vi "Calculate Desired States.vi"(8 "error in (no error)":errorcluster, 10 "Vessel In":refnum<class "Vessel.lvclass">, 11 "CJ Oculus Rift Guidance in":refnum<class "Oculus Rift Guidance.lvclass">) -> (0 "error out":errorcluster, 2 "Vessel Out":refnum<class "Vessel.lvclass">, 3 "CJ Oculus Rift Guidance out":refnum<class "Oculus Rift Guidance.lvclass">)   [LabVIEW 2014, in "Guidance Library.lvlib" / "Oculus Rift Guidance.lvclass"]
uses:
  Oculus Rift Guidance.lvclass
  ROV/Vessel.lvclass
  <vilib>/Analysis/Matrix/Datatypes/RealMatrix.ctl
  <vilib>/Analysis/baseanly.llb/A x Vector.vi
  Library/Kinematics/J_euler.vi
  Reference Models/Reference Model Joystick.vi
  Library/Integrator/Integrator trapez vector.vi
  Supervisor/Supervisor.lvclass
  <vilib>/Analysis/NI_AALBase.lvlib
  <vilib>/Analysis/Matrix/NI_Matrix.lvlib
panel:
  in  "Reset 0 Pos":bool
  in  "reset":bool
  in  "reset init pos":bool
  out "a 3":dbl(graph)
  out "a 2":dbl(graph)
  out "a":dbl(graph)
  in  "T 3":T1=[[0.0, -1.0, 0.0, 0.0, 0.0, 0.0], [-1.0, 0.0, 0.0, 0.0, 0.0, 0.0], [0.0, 0.0, 0.0, 0.0, 0.0, 0.0], [0.0, 0.0, 0.0, 0.0, 0.0, 0.0], [0.0, 0.0, 0.0, 0.0, 0.0, 0.0], [0.0, 0.0, 0.0, 0.0, 0.0, -1.0]]
  out "Nu_max":dbl[](array[numeric])
  out "yaw":cluster{"Numeric":dbl, dbl}(graph)
  out "sway":cluster{"Numeric":dbl, dbl}(graph)
  out "Surge":cluster{"Numeric":dbl, dbl}(graph)
  in  "Delta":T1=[[1.0, 0.0, 0.0, 0.0, 0.0, 0.0], [1.0, 0.0, 0.0, 0.0, 0.0, 0.0], [1.0, 0.0, 0.0, 0.0, 0.0, 0.0], [1.0, 0.0, 0.0, 0.0, 0.0, 0.0], [1.0, 0.0, 0.0, 0.0, 0.0, 0.0], [1.0, 0.0, 0.0, 0.0, 0.0, 0.0]]
  in  "Omega":T1=[[0.8, 0.0, 0.0, 0.0, 0.0, 0.0], [0.8, 0.0, 0.0, 0.0, 0.0, 0.0], [0.8, 0.0, 0.0, 0.0, 0.0, 0.0], [0.8, 0.0, 0.0, 0.0, 0.0, 0.0], [0.8, 0.0, 0.0, 0.0, 0.0, 0.0], [0.8, 0.0, 0.0, 0.0, 0.0, 0.0]]
  in  "OR Response":u16=1
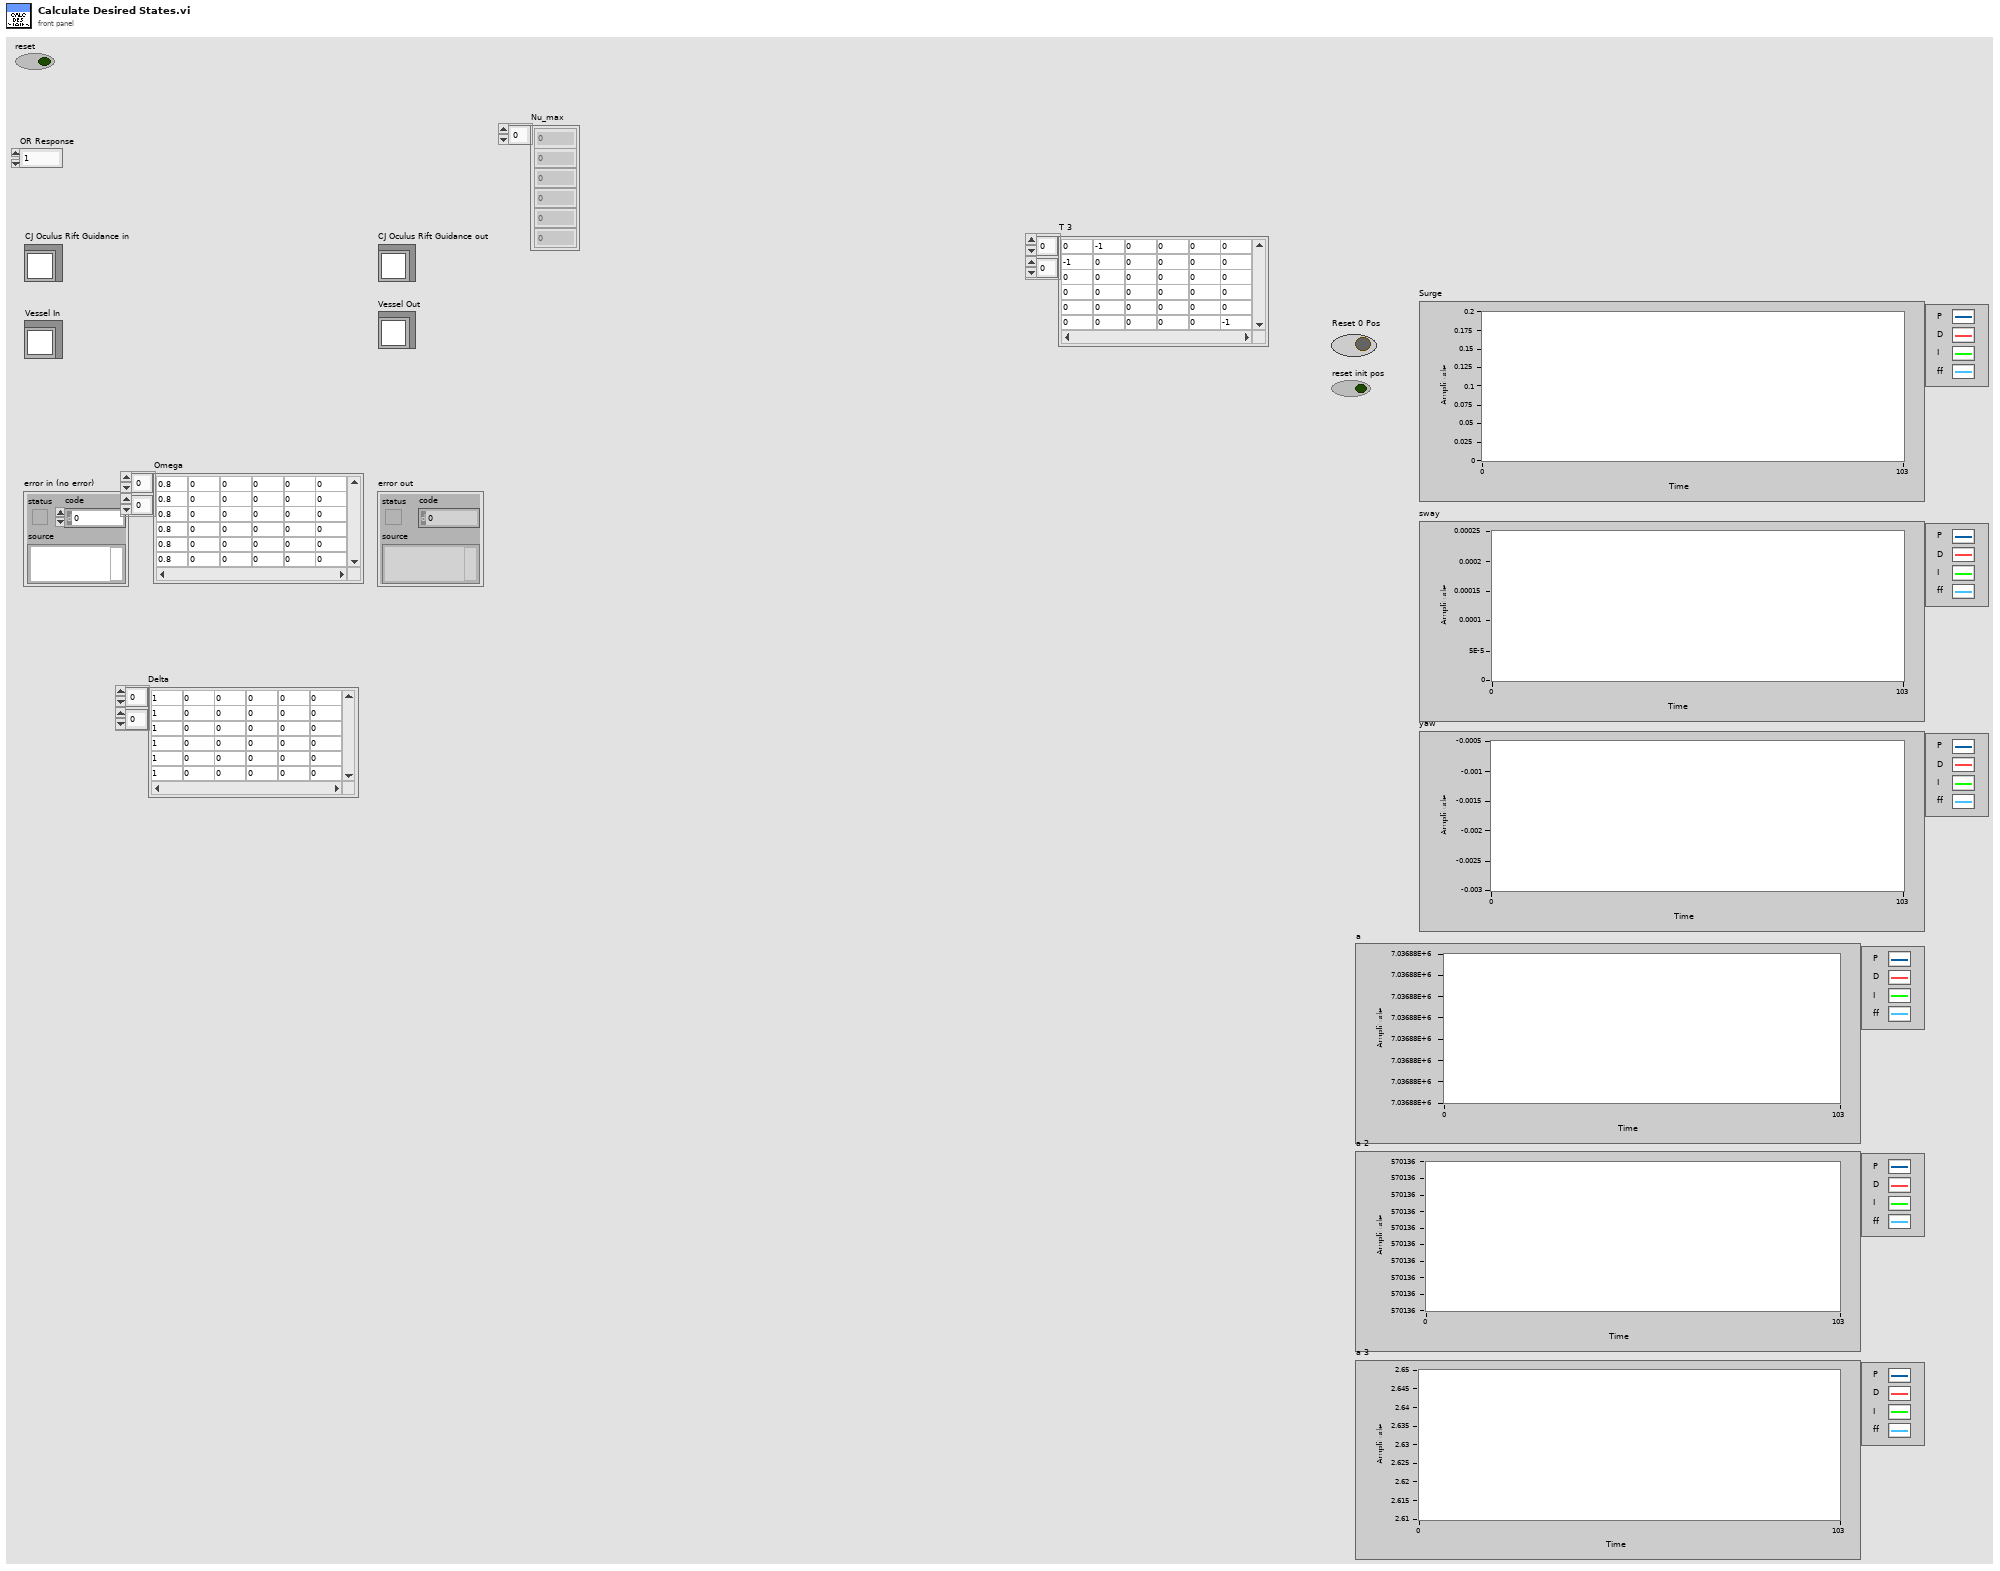
[diagram p1: front panel]
types:
  T1 = typedef "NI_Matrix.lvlib/RealMatrix.ctl" = dbl[][]
  T2 = cluster{"Measured":cluster{"Eta":dbl[], "Nu":dbl[], "Eta Dot":dbl[], "Nu Dot":dbl[]}, "Estimated":cluster{"Eta":dbl[], "Nu":dbl[], "Eta Dot":dbl[], "Nu Dot":dbl[]}, "Desired":cluster{"Eta":dbl[], "Nu":dbl[], "Eta Dot":dbl[], "Nu Dot":dbl[]}, "Previous Desired":cluster{"Eta":dbl[], "Nu":dbl[], "Eta Dot":dbl[], "Nu Dot":dbl[]}, "tau":dbl[], "Altitude":cluster{"Measured":dbl, "Estimated":dbl, "Desired":dbl, "Previous Desired":dbl, "Approximated":dbl, "grad F":dbl[]}, "rpm":dbl[], "Attitude":cluster{"Theta Measured":dbl[], "Theta Estimated":dbl[], "Omega Measured":dbl[], "Omega Estimated":dbl[], "Gyro Bias":dbl[]}}
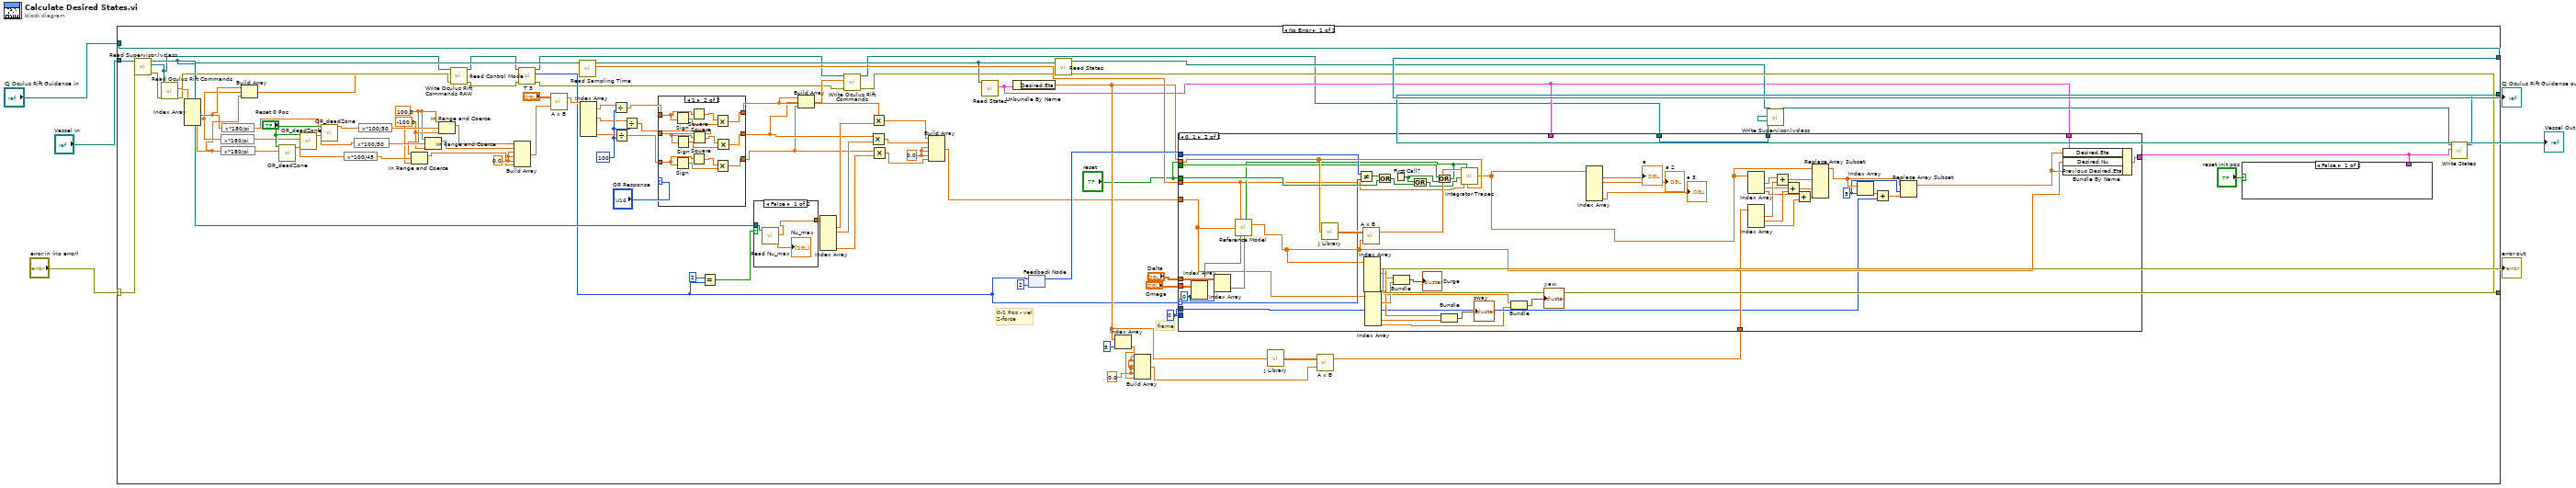
[diagram p0: block diagram]
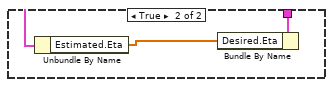
[diagram p2: hidden frame]
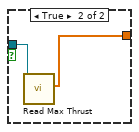
[diagram p3: hidden frame]
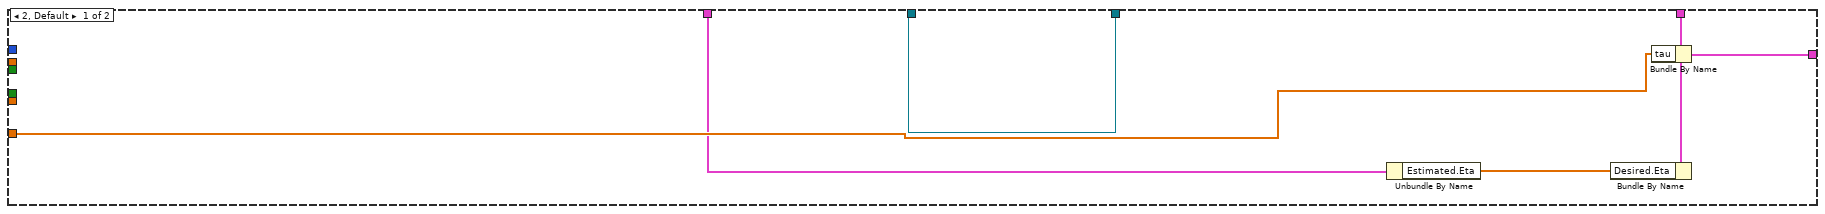
[diagram p4: hidden frame]
diagram:
  n1 = case shown="No Error" "error in (no error)" {
    selector: "error in (no error)" -> [w89 w172]
    tunnel: [w58 w172] -> w2
    tunnel: [w74 w171] -> w4
    tunnel: "CJ Oculus Rift Guidance in" -> [w74 w171]
    tunnel: "Vessel In" -> [w75 w170]
    tunnel: [w67 w170] -> w3
    frame No Error {
      w23 = 100.0 ("upper limit")
      w22 = -100.0 ("lower limit")
      w50 = 0.0
      w65 = 0.0 ("element")
      w66 = u16 0 ("Frame Mode")
      w82 = 0.0
      w88 = 100
      # "frame"
      # "0-1 Pos - vel\n2-force"
      n2 = call "Read Supervisor.lvclass.vi"("error in (no error)"=w89, "Vessel in"=w75) -> ("error out"=w90:errorcluster, "Supervisor.lvclass"=w16:refnum<class "Supervisor.lvclass">, "Vessel out"=w52:refnum<class "Vessel.lvclass">)  [unwired: 7 in]
      n3 = call-dynamic "Read Oculus Rift Commands.vi"("error in (no error)"=w90, "Supervisor in"=w16) -> ("error out"=w17:errorcluster, "Oculus Rift Commands"=w21:dbl[])  [unwired: 7 in, 1 out]
      n4 = Index Array(array=w21) -> (element #2=w9:dbl, element #3=w8:dbl, element #4=w7:dbl)  [unwired: 4 in, 1 out]
      n5 = expression code="x*180/pi"(w8) -> (w31:dbl)
      n6 = expression code="x*180/pi"(w7) -> (w30:dbl)
      n7 = expression code="x*180/pi"(w9) -> (w11:dbl)
      n8 = Build Array(w9, w8, w7) -> (w10:dbl[])
      n9 = call "OR_deadZone.vi"("x in"=w30, "Reset 0 Pos"="Reset 0 Pos") -> ("x out"=w28:dbl)  [unwired: 9 in]
      n10 = call "OR_deadZone.vi"("x in"=w31, "Reset 0 Pos"="Reset 0 Pos") -> ("x out"=w27:dbl)  [unwired: 9 in]
      n11 = call "OR_deadZone.vi"("x in"=w11, "Reset 0 Pos"="Reset 0 Pos") -> ("x out"=w29:dbl)  [unwired: 9 in]
      n12 = expression code="x*100/45"(w28) -> (w25:dbl)
      n13 = expression code="x*100/30"(w27) -> (w24:dbl)
      n14 = expression code="x*100/30"(w29) -> (w26:dbl)
      n15 = In Range and Coerce(upper limit=w23, x=w25, lower limit=w22) -> (coerced(x)=w18:dbl)  [unwired: 1 out]
      n16 = In Range and Coerce(upper limit=w23, x=w24, lower limit=w22) -> (coerced(x)=w19:dbl)  [unwired: 1 out]
      n17 = In Range and Coerce(upper limit=w23, x=w26, lower limit=w22) -> (coerced(x)=w20:dbl)  [unwired: 1 out]
      n18 = call-dynamic "Write Oculus Rift Commands RAW.vi"("error in (no error)"=w17, "Oculus Rift Commands RAW"=w10, "Supervisor in"=w16) -> ("error out"=w13:errorcluster, "Supervisor out"=w15:refnum<class "Supervisor.lvclass">)  [unwired: 7 in]
      n19 = Build Array(w20, w19, w50, w50, w50, w18) -> (w49:dbl[])
      n20 = call-dynamic "Read Control Mode.vi"("error in (no error)"=w13, "Supervisor in"=w15) -> ("error out"=w12:errorcluster, "Control Mode"=w40:u16, "Supervisor out"=w14:refnum<class "Supervisor.lvclass">)  [unwired: 7 in]
      n21 = call-poly <vilib>:"A x B.vi"("Vector"=w49, "A"="T 3") -> ("A x Vector"=w48:dbl[])  [unwired: 1 out]
      n22 = call-dynamic "Read Sampling Time.vi"("Vessel in"=w52) -> ("Sampling Time"=w69:dbl, "Vessel out"=w68:refnum<class "Vessel.lvclass">)  [unwired: 8 in, 1 out]
      n23 = Index Array(array=w48) -> (element #1=w47:dbl, element #2=w46:dbl, element #6=w45:dbl)  [unwired: 6 in, 3 out]
      n24 = Divide(x=w47, y=w88) -> (x/y=w87:dbl)
      n25 = Divide(x=w45, y=w88) -> (x/y=w85:dbl)
      n26 = Divide(x=w46, y=w88) -> (x/y=w86:dbl)
      n27 = case shown="1" "OR Response" {
        tunnel: w87 -> [w157 w163]
        tunnel: [w157 w162] -> w37
        tunnel: w86 -> [w156 w161]
        tunnel: [w156 w160] -> w36
        tunnel: w85 -> [w155 w159]
        tunnel: [w155 w158] -> w35
        frame 0, Default {
        }
        frame 1 {
          n28 = Sign(1:w163) -> (0:w164:dbl)
          n29 = Sign(1:w159) -> (0:w168:dbl)
          n30 = Sign(1:w161) -> (0:w167:dbl)
          n31 = Square(x=w163) -> (x^2=w165:dbl)
          n32 = Square(x=w159) -> (x^2=w169:dbl)
          n33 = Square(x=w161) -> (x^2=w166:dbl)
          n34 = Multiply(x=w165, y=w164) -> (x*y=w162:dbl)
          n35 = Multiply(x=w169, y=w168) -> (x*y=w158:dbl)
          n36 = Multiply(x=w166, y=w167) -> (x*y=w160:dbl)
        }
      }
      n37 = Equal?(x=u16 2, y=w40) -> (x = y?=w53:bool)
      n38 = case shown="False" w53 {
        tunnel: [w94 w96] -> w83
        tunnel: w52 -> [w93 w95]
        frame False {
          n39 = call "Read Nu_max.vi"("Vessel in"=w93) -> ("Nu_max"=w94:dbl[])  [unwired: 8 in, 2 out]
          "Nu_max" <- w94
        }
        frame True {
          n40 = call "Read Max Thrust.vi"("Vessel in"=w95) -> ("Max Thrust"=w96:dbl[])  [unwired: 8 in, 2 out]
        }
      }
      n41 = Build Array(w37, w36, w35) -> (w34:dbl[])
      n42 = Index Array(array=w83) -> (element #1=w80:dbl, element #2=w79:dbl, element #6=w78:dbl)  [unwired: 6 in, 3 out]
      n43 = call-dynamic "Write Oculus Rift Commands.vi"("error in (no error)"=w12, "Oculus Rift Commands"=w34, "Supervisor in"=w14) -> ("error out"=w33:errorcluster, "Supervisor out"=w38:refnum<class "Supervisor.lvclass">)  [unwired: 7 in]
      n44 = Multiply(x=w36, y=w79) -> (x*y=w77:dbl)
      n45 = Multiply(x=w37, y=w80) -> (x*y=w76:dbl)
      n46 = Multiply(x=w35, y=w78) -> (x*y=w81:dbl)
      n47 = Build Array(w76, w77, w82, w82, w82, w81) -> (w44:dbl[])
      n48 = call-dynamic "Read States.vi"("Vessel in"=w68) -> ("States"=w43:T2)  [unwired: 8 in, 2 out]
      n49 = Unbundle By Name(w43) -> ("Desired.Eta"=w60:dbl[])
      n50 = feedback-in #1(w40) -> ()
      n51 = feedback #1(u16 2 ("Control Mode")) -> (w70:u16)
      n52 = call-dynamic "Read States.vi"("error in (no error)"=w33, "Vessel in"=w68) -> ("error out"=w58:errorcluster, "Vessel out"=w55:refnum<class "Vessel.lvclass">)  [unwired: 7 in, 1 out]
      n53 = Index Array(array=w60, index=5) -> (element=w63:dbl)
      n54 = Build Array(w65, w65, w65, w65, w65, w63) -> (w62:dbl[])
      n55 = call-poly "J Library.vi"("eta"=w60) -> ("J"=w59:T1)
      n56 = call-poly <vilib>:"A x B.vi"("Vector"=w62, "A"=w59) -> ("A x Vector"=w61:dbl[])  [unwired: 1 out]
      n57 = case shown="0, 1" w40 {
        selector: w40 -> [_ w127]
        tunnel: w44 -> [w100 w117]
        tunnel: w60 -> [_ w141]
        tunnel: w69 -> [_ w107]
        tunnel: "Delta" -> [_ w154]
        tunnel: "Omega" -> [_ w153]
        tunnel: w61 -> [_ w152]
        tunnel: w66 -> [_ w110]
        tunnel: w66 -> [_ _]
        tunnel: "reset" -> [_ w125]
        tunnel: "reset" -> [_ w128]
        tunnel: [w102 w122] -> w42
        tunnel: w70 -> [_ w126]
        tunnel: w43 -> [w99 w121]
        tunnel: w38 -> [w101 w120]
        tunnel: [w101 w120] -> w57
        tunnel: w43 -> [w97 _]
        frame 2, Default {
          n58 = Unbundle By Name(w97) -> ("Estimated.Eta"=w98:dbl[])
          n59 = Bundle By Name(cluster=w99, "Desired.Eta"=w98) -> ()  [unwired: 1 out]
          n60 = Bundle By Name(cluster=w99, "tau"=w100) -> (w102:T2)
        }
        frame 0, 1 {
          w132 = 5 ("index")
          w139 = 0
          n61 = Index Array(array=w153, index (col)=w139) -> (element=w138:dbl[])  [unwired: 1 in]
          n62 = Index Array(array=w154, index (col)=w139) -> (element=w137:dbl[])  [unwired: 1 in]
          n63 = call-poly "J Library.vi"("eta"=w141) -> ("J"=w135:T1)
          n64 = Not Equal?(x=w126, y=w127) -> (x != y?=w129:bool)
          n65 = Index Array(array=w117) -> (element #1=w115:dbl, element #2=w112:dbl, element #6=w108:dbl)  [unwired: 6 in, 3 out]
          n66 = Or(x=w129, y=w128) -> (x .or. y?=w130:bool)
          n67 = First Call?() -> (First Call?: T/F=w131:bool)
          n68 = Or(x=w131, y=w130) -> (x .or. y?=w124:bool)
          n69 = Or(x=w125, y=w131) -> (x .or. y?=w123:bool)
          n70 = call-poly "Reference Model.vi"("dt"=w107, "Reset"=w123, "Reference Joystick"=w117, "Omega"=w138, "Delta"=w137) -> ("nu_desired"=w118:dbl[])  [unwired: 9 in, 1 out]
          n71 = call-poly <vilib>:"A x B.vi"("Vector"=w118, "A"=w135) -> ("A x Vector"=w140:dbl[])  [unwired: 1 out]
          n72 = Index Array(array=w118) -> (element #1=w116:dbl, element #2=w113:dbl, element #6=w109:dbl)  [unwired: 6 in, 3 out]
          n73 = Bundle("Numeric"=w116, w115) -> (→"Surge":cluster{"Numeric":dbl, dbl})  [unwired: 1 in]
          n74 = Bundle("Numeric"=w113, w112) -> (→"sway":cluster{"Numeric":dbl, dbl})  [unwired: 1 in]
          n75 = call-poly "Integrator Trapez.vi"("IC"=w141, "Reset"=w123, "dt"=w107, "Initialize"=w124, "Input"=w140) -> ("Output"=w106:dbl[])  [unwired: 1 in]
          n76 = Bundle("Numeric"=w109, w108) -> (→"yaw":cluster{"Numeric":dbl, dbl})  [unwired: 1 in]
          n77 = Index Array(array=w106) -> (element #1=→"a":dbl, element #2=→"a 2":dbl, element #6=→"a 3":dbl)  [unwired: 6 in, 3 out]
          n78 = Index Array(array=w106) -> (element #1=w145:dbl, element #2=w144:dbl, element #3=w143:dbl)  [unwired: 3 in]
          n79 = Index Array(array=w152) -> (element #1=w148:dbl, element #2=w147:dbl, element #3=w146:dbl)  [unwired: 3 in]
          n80 = Add(x=w145, y=w148) -> (x+y=w151:dbl)
          n81 = Add(x=w144, y=w147) -> (x+y=w150:dbl)
          n82 = Add(x=w143, y=w146) -> (x+y=w149:dbl)
          n83 = Replace Array Subset(array=w106, new element #1=w151, new element #2=w150, new element #3=w149) -> (w142:dbl[])  [unwired: 3 in]
          n84 = Index Array(array=w142, index=w132) -> (element=w134:dbl)
          n85 = Add(x=w134, y=w110) -> (x+y=w133:dbl)
          n86 = Replace Array Subset(array=w142, new element=w133, index=w132) -> (w136:dbl[])
          n87 = Bundle By Name(cluster=w121, "Desired.Eta"=w136, "Desired.Nu"=w118, "Previous Desired.Eta"=w136) -> (w122:T2)
        }
      }
      n88 = call "Write Supervisor.lvclass.vi"("Supervisor.lvclass"=w57, "Vessel in"=w55) -> ("Vessel out"=w56:refnum<class "Vessel.lvclass">)  [unwired: 8 in, 1 out]
      n89 = case shown="False" "reset init pos" {
        tunnel: w42 -> [_ w92]
        frame False {
        }
        frame True {
          n90 = Unbundle By Name(w92) -> ("Estimated.Eta"=w91:dbl[])
          n91 = Bundle By Name(cluster=w92, "Desired.Eta"=w91) -> ()  [unwired: 1 out]
        }
      }
      n92 = call-dynamic "Write States.vi"("States"=w42, "Vessel in"=w56) -> ("Vessel out"=w67:refnum<class "Vessel.lvclass">)  [unwired: 8 in, 1 out]
    }
    frame Error {
    }
  }
  "error out" <- w2
  "CJ Oculus Rift Guidance out" <- w4
  "Vessel Out" <- w3
